vi "Write SA Pin.vi"(8 "error in (no error)":errorcluster, 10 "SA Pin":string, 11 "LTE_ACP in":refnum<class "LTE_ACP.lvclass">=refnum) -> (0 "error out":errorcluster, 3 "LTE_ACP out":refnum<class "LTE_ACP.lvclass">)   [LabVIEW 2016, in "SeqAuto Evaluations.lvlib" / "LTE_ACP.lvclass"]
uses:
  LTE_ACP.lvclass
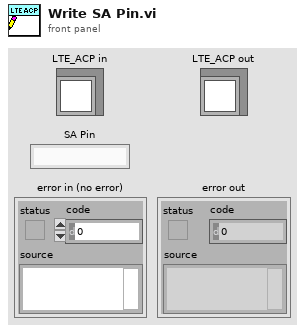
[diagram p1: front panel]
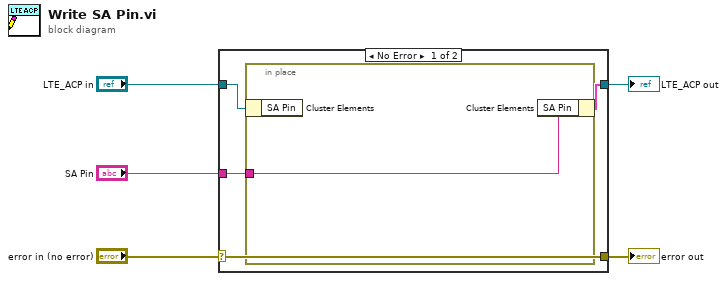
[diagram p0: block diagram]
diagram:
  n1 = case shown="No Error" "error in (no error)" {
    selector: "error in (no error)" -> [w9 w11]
    tunnel: [w9 w11] -> w4
    tunnel: [w6 w12] -> w2
    tunnel: "LTE_ACP in" -> [w7 w12]
    tunnel: "SA Pin" -> [w8 _]
    frame No Error {
      n2 = in-place {
        in-place-border: w8 -> [w10]
        n3 = in-place-cluster #1(w7) -> ()  [unwired: 1 out]
        n4 = in-place-cluster #1("SA Pin"=w10) -> (w6:cluster{})
      }
    }
    frame Error {
    }
  }
  "error out" <- w4
  "LTE_ACP out" <- w2
